vi "clases.vi"() -> ()   [LabVIEW 2016]
panel:
  in  "Enum":T1(ring)
  out "String":string
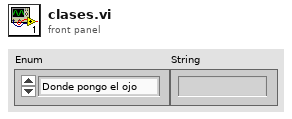
[diagram p1: front panel]
types:
  T1 = enum16{"Donde pongo el ojo", "No importa lo grueso"}
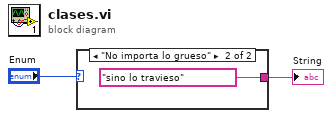
[diagram p0: block diagram]
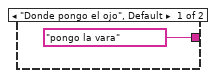
[diagram p2: hidden frame]
diagram:
  n1 = case shown="\"No importa lo grueso\"" "Enum" {
    tunnel: ["pongo la vara" "sino lo travieso"] -> w1
    frame "Donde pongo el ojo", Default {
    }
    frame "No importa lo grueso" {
    }
  }
  "String" <- w1
